vi "FGV PNS Steuerung.vi"(6 "Enum":enum16{"initialisieren", "lesen", "schreiben"}(ring), 11 "Steuerung PNS (Eingang)":refnum<class "Steuerung PNS.lvclass">) -> (3 "Steuerung PNS (Ausgang)":refnum<class "Steuerung PNS.lvclass">)   [LabVIEW 2020]
doc: "FGV um Objektreferenzen in mehreren VIs nutzen zu können.\nBeim Initialisieren wird eine Objektinstanz erzeugt.\nNach dem Wechsel auf eine spezifische SubKlasse muss diese wieder in dieses FGV geschrieben werden.\n\nNach jeder Datenänderung muss ebenfalls die neue Objektreferenz hier her zurück geschrieben werden,\nsonst ist kein Zugriff auf diese neuen oder geänderten Daten möglich !\nRIW"
uses:
  Steuerung PNS.lvclass
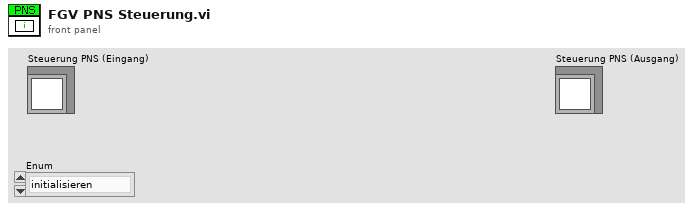
[diagram p1: front panel]
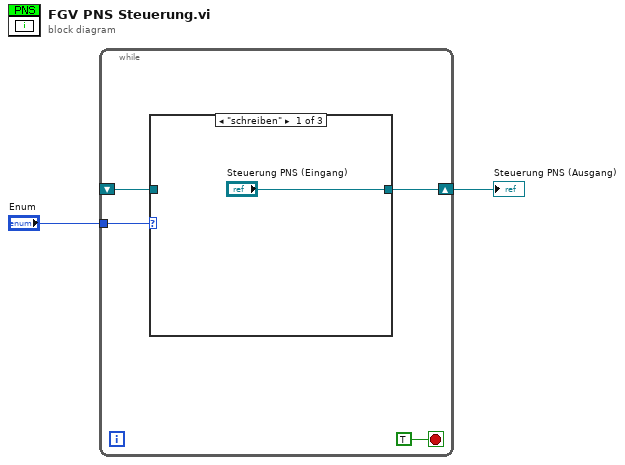
[diagram p0: block diagram]
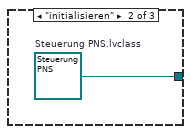
[diagram p2: hidden frame]
diagram:
  n1 = while {
    shift-right: [w5] -> w1
    shift-left: _ -> [w4]
    tunnel: "Enum" -> [w3]
    stop <- TRUE stop-if-true
    n2 = case shown="\"schreiben\"" w3 {
      tunnel: w4 -> [_ _ w9]
      tunnel: ["Steuerung PNS (Eingang)" w8 w9] -> w5
      frame "schreiben" {
      }
      frame "initialisieren" {
        w8 = refnum<class "Steuerung PNS.lvclass"> refnum  # Steuerung PNS.lvclass
      }
      frame "lesen", Default {
      }
    }
  }
  "Steuerung PNS (Ausgang)" <- w1
